vi "defer panel updates.vi"(7 "Defer Panel Updates ? (T)":bool=TRUE, 8 "Error in":errorcluster, 10 "VI Path in":path, 11 "VI ref in":refnum<vi>) -> (0 "Error out":errorcluster)   [LabVIEW 2023, in "Reusable Library.lvlib"]
doc: "This VI defers the front panel updates when \"Defer Panel Updates?\" terminal is true and vice versa. VI Ref or VI path any one is enough, if both the terminals are unwired defaultly it takes the ref of the current vi where this sub vi is kept."
uses:
  Reusable Library.lvlib
panel:
  # "Samuel J\n     Measurement Engineer\n     Certified LabVIEW Architect\n     Vestas Technology R&D Chennai"
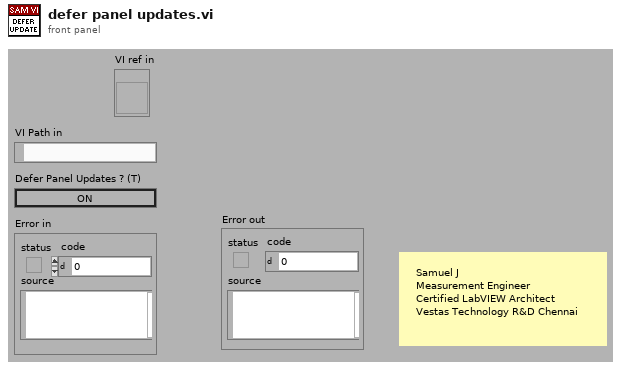
[diagram p1: front panel]
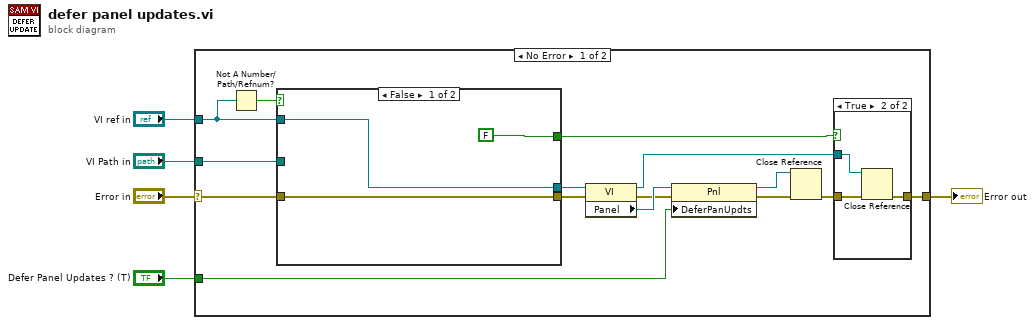
[diagram p0: block diagram]
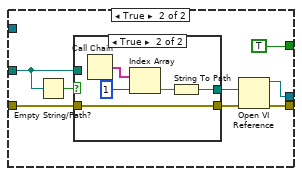
[diagram p3: hidden frame]
diagram:
  n1 = case shown="No Error" "Error in" {
    selector: "Error in" -> [w12 w43]
    tunnel: "Defer Panel Updates ? (T)" -> [w19 _]
    tunnel: [w8 w43] -> w4
    tunnel: "VI Path in" -> [w15 _]
    tunnel: "VI ref in" -> [w13 _]
    frame No Error {
      n2 = Not A Number/Path/Refnum?(number/path/refnum=w13) -> (NaN/Path/Refnum?=w14:bool)
      n3 = case shown="False" w14 {
        tunnel: [w26 w35] -> w17
        tunnel: [w27 w34] -> w16
        tunnel: w15 -> [_ w31]
        tunnel: w12 -> [w27 w29]
        tunnel: w13 -> [w26 _]
        tunnel: [FALSE ("Boolean") TRUE ("Boolean")] -> w6
        frame False {
        }
        frame True {
          n4 = Empty String/Path?(string/path=w31) -> (empty?=w32:bool)
          n5 = case shown="True" w32 {
            tunnel: [w37 w39] -> w33
            tunnel: w31 -> [w37 _]
            tunnel: [w36 w38] -> w30
            tunnel: w29 -> [w36 w38]
            frame False {
            }
            frame True {
              n6 = Call Chain() -> (call chain=w42:string[])
              n7 = Index Array(array=w42, index=1) -> (element=w40:string)
              n8 = String To Path(string=w40) -> (path=w39:path)
            }
          }
          n9 = Open VI Reference(vi path=w33, error in (no error)=w30) -> (vi reference=w35:refnum<vi>, error out=w34:errorcluster)  [unwired: 4 out]
        }
      }
      n10 = property class="VI"(reference=w17, error in=w16) -> (reference out=w7:refnum<vi>, error out=w18:errorcluster, "Panel"=w20:refnum<vi>)
      n11 = property class="Pnl"(reference=w20, error in=w18, "DeferPanUpdts"=w19) -> (reference out=w11:refnum<vi>, error out=w10:errorcluster)
      n12 = Close Reference(reference=w11, error in (no error)=w10) -> (error out=w9:errorcluster)
      n13 = case shown="True" w6 {
        tunnel: w9 -> [w21 w24]
        tunnel: [w21 w23] -> w8
        tunnel: w7 -> [_ w22]
        frame False {
        }
        frame True {
          n14 = Close Reference(reference=w22, error in (no error)=w24) -> (error out=w23:errorcluster)
        }
      }
    }
    frame Error {
    }
  }
  "Error out" <- w4
